vi "Test Caller Called.vi"() -> ()   [LabVIEW 2020, in "CallerCalledTests.lvlib"]
uses:
  CallerCalledTests.lvlib
  <vilib>/addons/_JKI Toolkits/Caraya/classes/Test Suite/Define Test Suite (JUnit Report).vi
  <vilib>/SLL Drona/APIs/Stimulus/VI/MakeVIFrontMost.vi
  <vilib>/SLL Drona/APIs/Stimulus/ControlValue/ValueSignalByPathString.vi
  <vilib>/SLL Drona/APIs/Stimulus/ControlValue/ValueSignalLatchBooleanString.vi
  <vilib>/SLL Drona/APIs/Get/GetVI/GetVIByName.vi
  <vilib>/SLL Drona/APIs/Assert/AssertVI/AssertVIExecRunning.vi
  <vilib>/addons/_JKI Toolkits/Caraya/classes/Assert/Assert Equal Value_Variant.vi
  <vilib>/SLL Drona/APIs/Assert/AssertVI/AssertVIExecIdle.vi
  <vilib>/SLL Drona/APIs/Stimulus/VI/CloseVI.vi
  <vilib>/Utility/error.llb/Error Cluster From Error Code.vi
  <vilib>/ErrorRing/Error Ring.xnode
  <vilib>/addons/_JKI Toolkits/Caraya/classes/Test Suite/Test Suite.lvclass
  <vilib>/addons/_JKI Toolkits/Caraya/classes/Test/Test.lvclass
  <vilib>/SLL Drona/Drona.lvlib
  <vilib>/Wiresmith Technology/G CLI/CLI Class/CLI.lvclass
  <vilib>/SLL Drona/APIs/Stimulus/ControlValue/ControlValue.lvlib
  <vilib>/addons/_JKI Toolkits/Caraya/classes/Assert/Assert.lvclass
  <vilib>/SLL Drona/APIs/Assert/AssertVI/AssertVI.lvlib
  <vilib>/SLL Drona/APIs/Stimulus/VI/VI.lvlib
  <vilib>/SLL Drona/APIs/Get/GetVI/GetVI.lvlib
panel:
  out "Error out":errorcluster
  in  "Error in":errorcluster
  # "CALLER CALLED TEST"
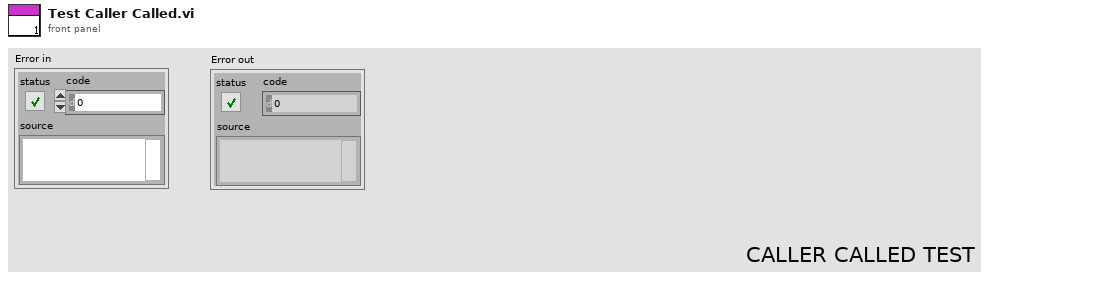
[diagram p1: front panel]
types:
  T1 = enum32{"Invalid", "Default", "Floating", "Floating/Auto-Hide", "Modal"}
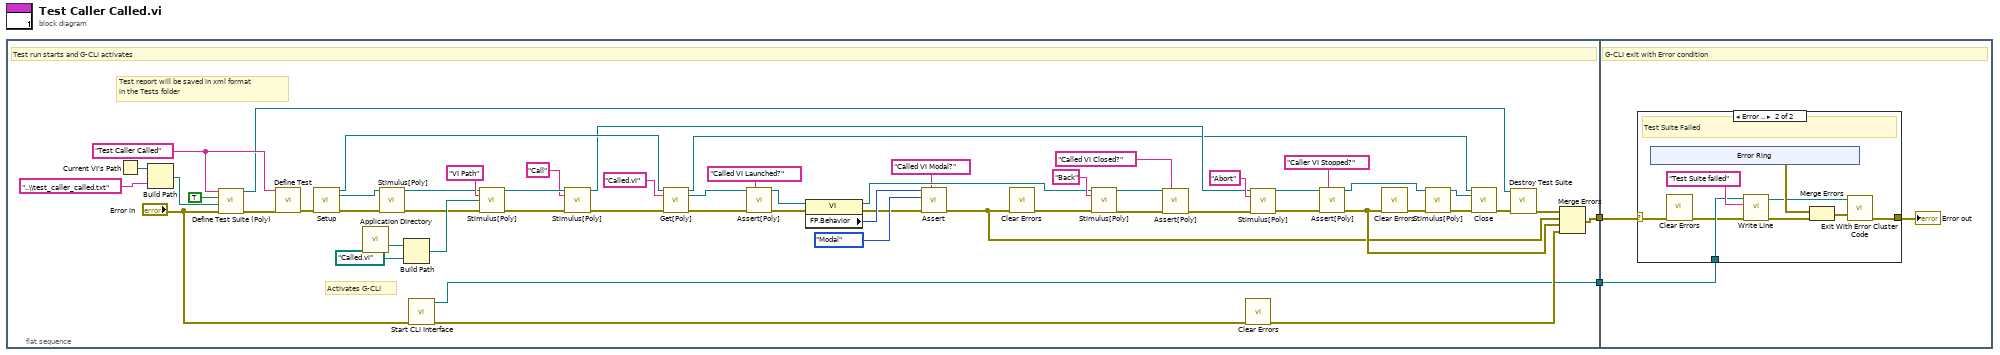
[diagram p0: block diagram]
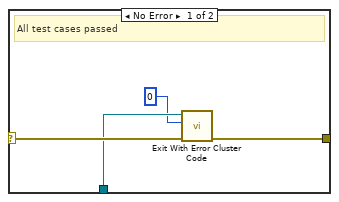
[diagram p2: hidden frame]
diagram:
  n1 = flat-sequence {
    tunnel: [w39] -> w2
    tunnel: [w38] -> w1
    tunnel: w2 -> [w62]
    tunnel: w1 -> [w61]
    frame #0 {
      w51 = "Test Caller Called" ("Label (VI Title)")
      # "Activates G-CLI"
      # "Test report will be saved in xml format\nin the Tests folder"
      # "Test run starts and G-CLI activates"
      n2 = Current VI's Path() -> (path=w50:path)
      n3 = Build Path(base path=w50, name or relative path="..\\test_caller_called.txt") -> (appended path=w48:path)
      n4 = call-poly <vilib>:"Define Test Suite (Poly).vi"("error in (no error)"="Error in", "Report Path"=w48, "Interactive"=TRUE, "Label (VI Title)"=w51) -> ("error out"=w52:errorcluster, "Test Suite"=w45:refnum<class "Test Suite.lvclass">)  [unwired: 5 in, 1 out]
      n5 = call <vilib>:"Define Test.vi"("error in (no error)"=w52, "Label (VI Title)"=w51) -> ("error out"=w59:errorcluster)  [unwired: 8 in, 1 out]
      n6 = call <vilib>:"Setup.vi"("error in"=w59) -> ("Application Ref"=w34:refnum<vi>, "VI Reference Out"=w4:refnum<vi>, "error out"=w58:errorcluster)  [unwired: 12 in]
      n7 = call <vilib>:"Application Directory.vi"() -> ("Application Directory"=w37:path)
      n8 = call-poly <vilib>:"Stimulus[Poly].vi"("VI Reference In"=w4, "error in"=w58) -> ("VI Reference Out"=w3:refnum<vi>, "error out"=w5:errorcluster)  [unwired: 12 in]
      n9 = Build Path(base path=w37, name or relative path=path "Called.vi") -> (appended path=w55:path)
      n10 = call <vilib>:"Start CLI Interface.vi"("error in (no error)"="Error in") -> ("error out"=w41:errorcluster, "CLI out"=w38:refnum<class "CLI.lvclass">)  [unwired: 7 in, 2 out]
      n11 = call-poly <vilib>:"Stimulus[Poly].vi"("VI Reference In"=w3, "Control Path"="VI Path", "Value (Signaling)"=w55, "error in"=w5) -> ("VI Reference Out"=w36:refnum<vi>, "error out"=w35:errorcluster)  [unwired: 10 in]
      n12 = call-poly <vilib>:"Stimulus[Poly].vi"("VI Reference In"=w36, "Control Path"="Call", "error in"=w35) -> ("VI Reference Out"=w15:refnum<vi>, "error out"=w30:errorcluster)  [unwired: 11 in]
      n13 = call-poly <vilib>:"Get[Poly].vi"("Application Ref in"=w34, "VI Name"="Called.vi", "error in (no error)"=w30) -> ("Application Ref out"=w14:refnum<vi>, "VI Reference"=w29:refnum<vi>, "error out"=w28:errorcluster)  [unwired: 10 in]
      n14 = call-poly <vilib>:"Assert[Poly].vi"("VI Reference In"=w29, "Test Label"="Called VI Launched?", "Error In"=w28) -> ("VI Reference Out"=w18:refnum<vi>, "Error Out"=w20:errorcluster)  [unwired: 11 in]
      n15 = property on="Property Node" class="VI"(reference=w18, error in=w20) -> (reference out=w17:refnum<vi>, error out=w19:errorcluster, "FP.Behavior"=w22:T1)
      n16 = call-poly <vilib>:"Assert.vi"("Label"="Called VI Modal?" ("Test Label"), "error in (no error)"=w19, "Y"=T1."Modal" ("Front Panel Window:Behavior"), "X"=w22) -> ("error out"=w6:errorcluster)  [unwired: 6 in, 1 out]
      n17 = call <vilib>:"Clear Errors.vi"("error in (no error)"=w6) -> ("error out"=w7:errorcluster)  [unwired: 5 in, 1 out]
      n18 = call-poly <vilib>:"Stimulus[Poly].vi"("VI Reference In"=w17, "Control Path"="Back", "error in"=w7) -> ("VI Reference Out"=w24:refnum<vi>, "error out"=w23:errorcluster)  [unwired: 11 in]
      n19 = call-poly <vilib>:"Assert[Poly].vi"("VI Reference In"=w24, "Test Label"="Called VI Closed?", "Error In"=w23) -> ("Error Out"=w13:errorcluster)  [unwired: 11 in, 1 out]
      n20 = call <vilib>:"Clear Errors.vi"("error in (no error)"=w41) -> ("error out"=w40:errorcluster)  [unwired: 5 in, 1 out]
      n21 = call-poly <vilib>:"Stimulus[Poly].vi"("VI Reference In"=w15, "Control Path"="Abort", "error in"=w13) -> ("VI Reference Out"=w12:refnum<vi>, "error out"=w11:errorcluster)  [unwired: 11 in]
      n22 = call-poly <vilib>:"Assert[Poly].vi"("VI Reference In"=w12, "Test Label"="Caller VI Stopped?", "Error In"=w11) -> ("VI Reference Out"=w8:refnum<vi>, "Error Out"=w9:errorcluster)  [unwired: 11 in]
      n23 = call <vilib>:"Clear Errors.vi"("error in (no error)"=w9) -> ("error out"=w42:errorcluster)  [unwired: 5 in, 1 out]
      n24 = call-poly <vilib>:"Stimulus[Poly].vi"("VI Reference In"=w8, "error in"=w42) -> ("VI Reference Out"=w54:refnum<vi>, "error out"=w53:errorcluster)  [unwired: 12 in]
      n25 = call <vilib>:"Close.vi"("Application Ref"=w14, "VI Reference"=w54, "error in"=w53) -> ("error out"=w46:errorcluster)  [unwired: 12 in]
      n26 = call-dynamic "Destroy Test Suite.vi"("error in (no error)"=w46, "Test Suite in"=w45) -> ("error out"=w43:errorcluster)  [unwired: 8 in, 1 out]
      n27 = Merge Errors(w43, w6, w9, w40) -> (w39:errorcluster)
    }
    frame #1 {
      # "G-CLI exit with Error condition"
      n28 = case shown="Error .." w62 {
        selector: w62 -> [w66 w70]
        tunnel: w61 -> [w65 w68]
        tunnel: [w63 w75] -> w60
        frame No Error {
          # "All test cases passed"
          n29 = call <vilib>:"Exit With Error Cluster Code.vi"("error in (no error)"=w66, "No Error Code (0)"=0, "CLI in"=w65) -> ("error out"=w63:errorcluster)  [unwired: 8 in]
        }
        frame Error {
          # "Test Suite Failed"
          n30 = xnode ("Error Ring")() -> ("error out"=w72:errorcluster)
          n31 = call <vilib>:"Clear Errors.vi"("error in (no error)"=w70) -> ("error out"=w67:errorcluster)  [unwired: 5 in, 1 out]
          n32 = call <vilib>:"Write Line.vi"("error in (no error)"=w67, "Text to Write"="Test Suite failed", "CLI in"=w68) -> ("error out"=w71:errorcluster, "CLI out"=w69:refnum<class "CLI.lvclass">)  [unwired: 7 in]
          n33 = Merge Errors(w72, w71) -> (w73:errorcluster)
          n34 = call <vilib>:"Exit With Error Cluster Code.vi"("error in (no error)"=w73, "CLI in"=w69) -> ("error out"=w75:errorcluster)  [unwired: 9 in]
        }
      }
      "Error out" <- w60
    }
  }
